vi "stage_control.vi"() -> ()   [LabVIEW 2009]
uses:
  global_stage_initialised.vi
  <vilib>/Utility/inputDevices.llb/joystickAcquire.vi
  <vilib>/Utility/inputDevices.llb/closeJoystick.vi
panel:
  in  "Joystick Index":i32
  in  "SN von Controller 1":string="0135500571"
  in  "Position auslesen":bool
  out "Joystickauslese":T1(ring)
  out "X-Achse pos/neg fahren":i32 min=-3000 max=2000
  out "Y-Achse pos/neg fahren":i32 min=-3000 max=2000
  in  "Schrittweite verringern":bool
  in  "Schrittweite erhoehen":bool
  out "Z-Achse pos fahren":bool
  out "Z-Achse neg fahren":bool
  out "Joystick ID":refnum<k1> caption="Geräte-ID"
  out "z-Achse":i32
  out "y-Achse":i32
  out "x-Achse":i32
  in  "Schrittweite [µm]":u16(ring) items=["500,0", "200,0", "100,0", "50,0", "20,0", "10,0", "5,0", "2,0", "1,0", "0,5", "0,1"]
  out "Aktuelle xyz-Position [mm]":dbl[](array[numeric]) format="%.5g"
  in  "Geschwindigkeit einstellen":bool
  in  "Ziel Geschwindigkeit [mm/s]":dbl=0.3 min=0.01 max=0.6 step=0.001 format="%.3g"
  out "Geschwindigkeit [mm/s]":dbl format="%.3g"
  in  "Negativer Schritt":bool[](array[boolean])
  in  "Positiver Schritt":bool[](array[boolean])
  out "error out":errorcluster
  out "Achse in \nBewegung":bool
  in  "Ziel xyz-Position [mm]":dbl[](array[numeric]) step=1e-05 format="%.5g"
  out "xyz-Bezeichnung":string[](array[string])=["x [mm]", "y [mm]", "z [mm]"]
  in  "Bühnen schließen":bool
  out "Bühnen\ninitialisiert":bool
  # "Steuerung der 3D-Translationsbühne von PI"
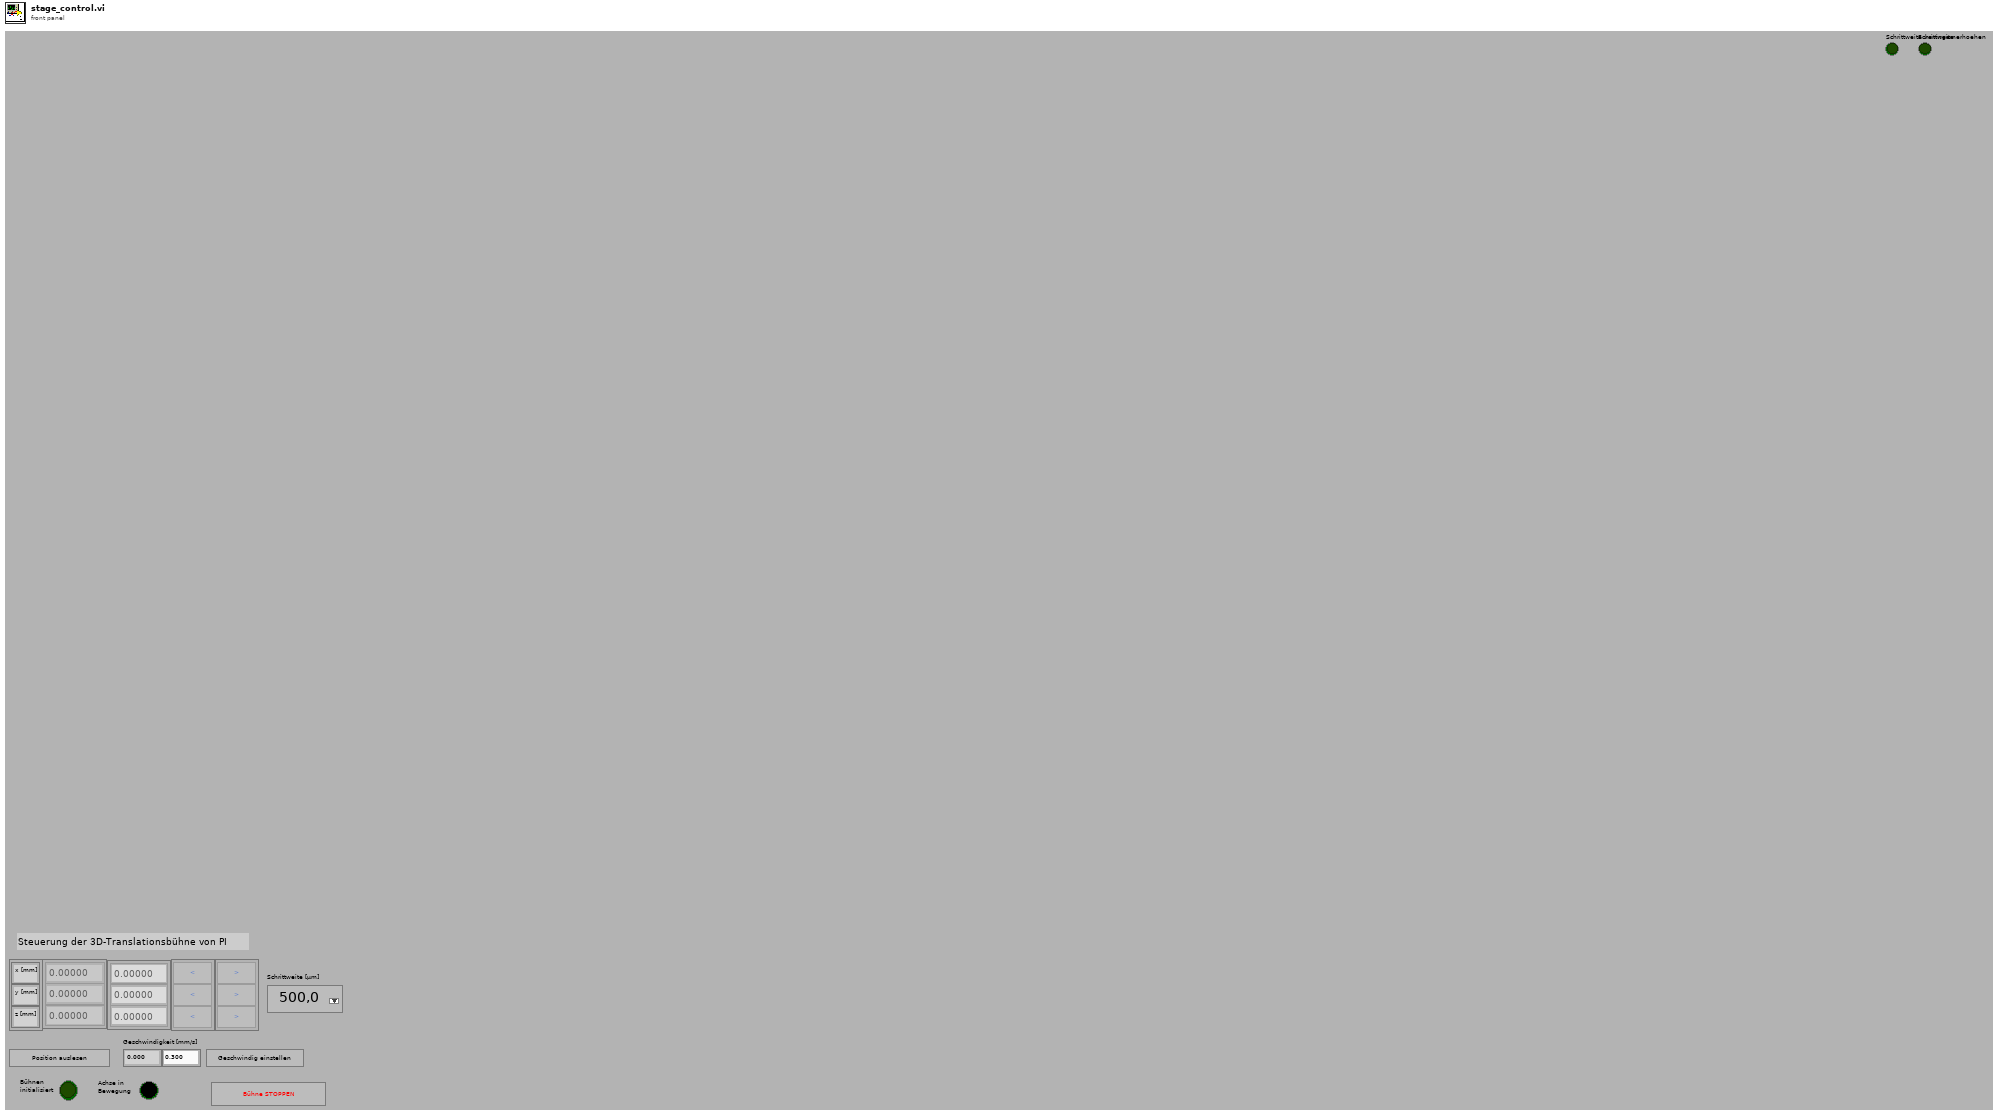
[diagram p1: front panel]
types:
  T1 = enum16{"Nichts tun", "X-Achse", "Y-Achse", "Z-Achse positiv", "Z-Achse negativ", "Schrittweite erhoehen", "Schrittweite verringern"}
  T2 = cluster{"X axis":i32, "Y axis":i32, "Z axis":i32, "X axis rotation":i32, "Y axis rotation":i32, "Z axis rotation":i32, "U axis":i32, "V axis":i32}
  T3 = cluster{"button 1":bool, "button 2":bool, "button 3":bool, "button 4":bool, "button 5":bool, "button 6":bool, "button 7":bool, "button 8":bool, "button 9":bool, "button 10":bool, "button 11":bool, "button 12":bool, "button 13":bool, "button 14":bool, "button 15":bool, "button 16":bool, "button 17":bool, "button 18":bool, "button 19":bool, "button 20":bool, "button 21":bool, "button 22":bool, "button 23":bool, "button 24":bool, "button 25":bool, "button 26":bool, "button 27":bool, "button 28":bool, "button 29":bool, "button 30":bool, "button 31":bool, "button 32":bool}
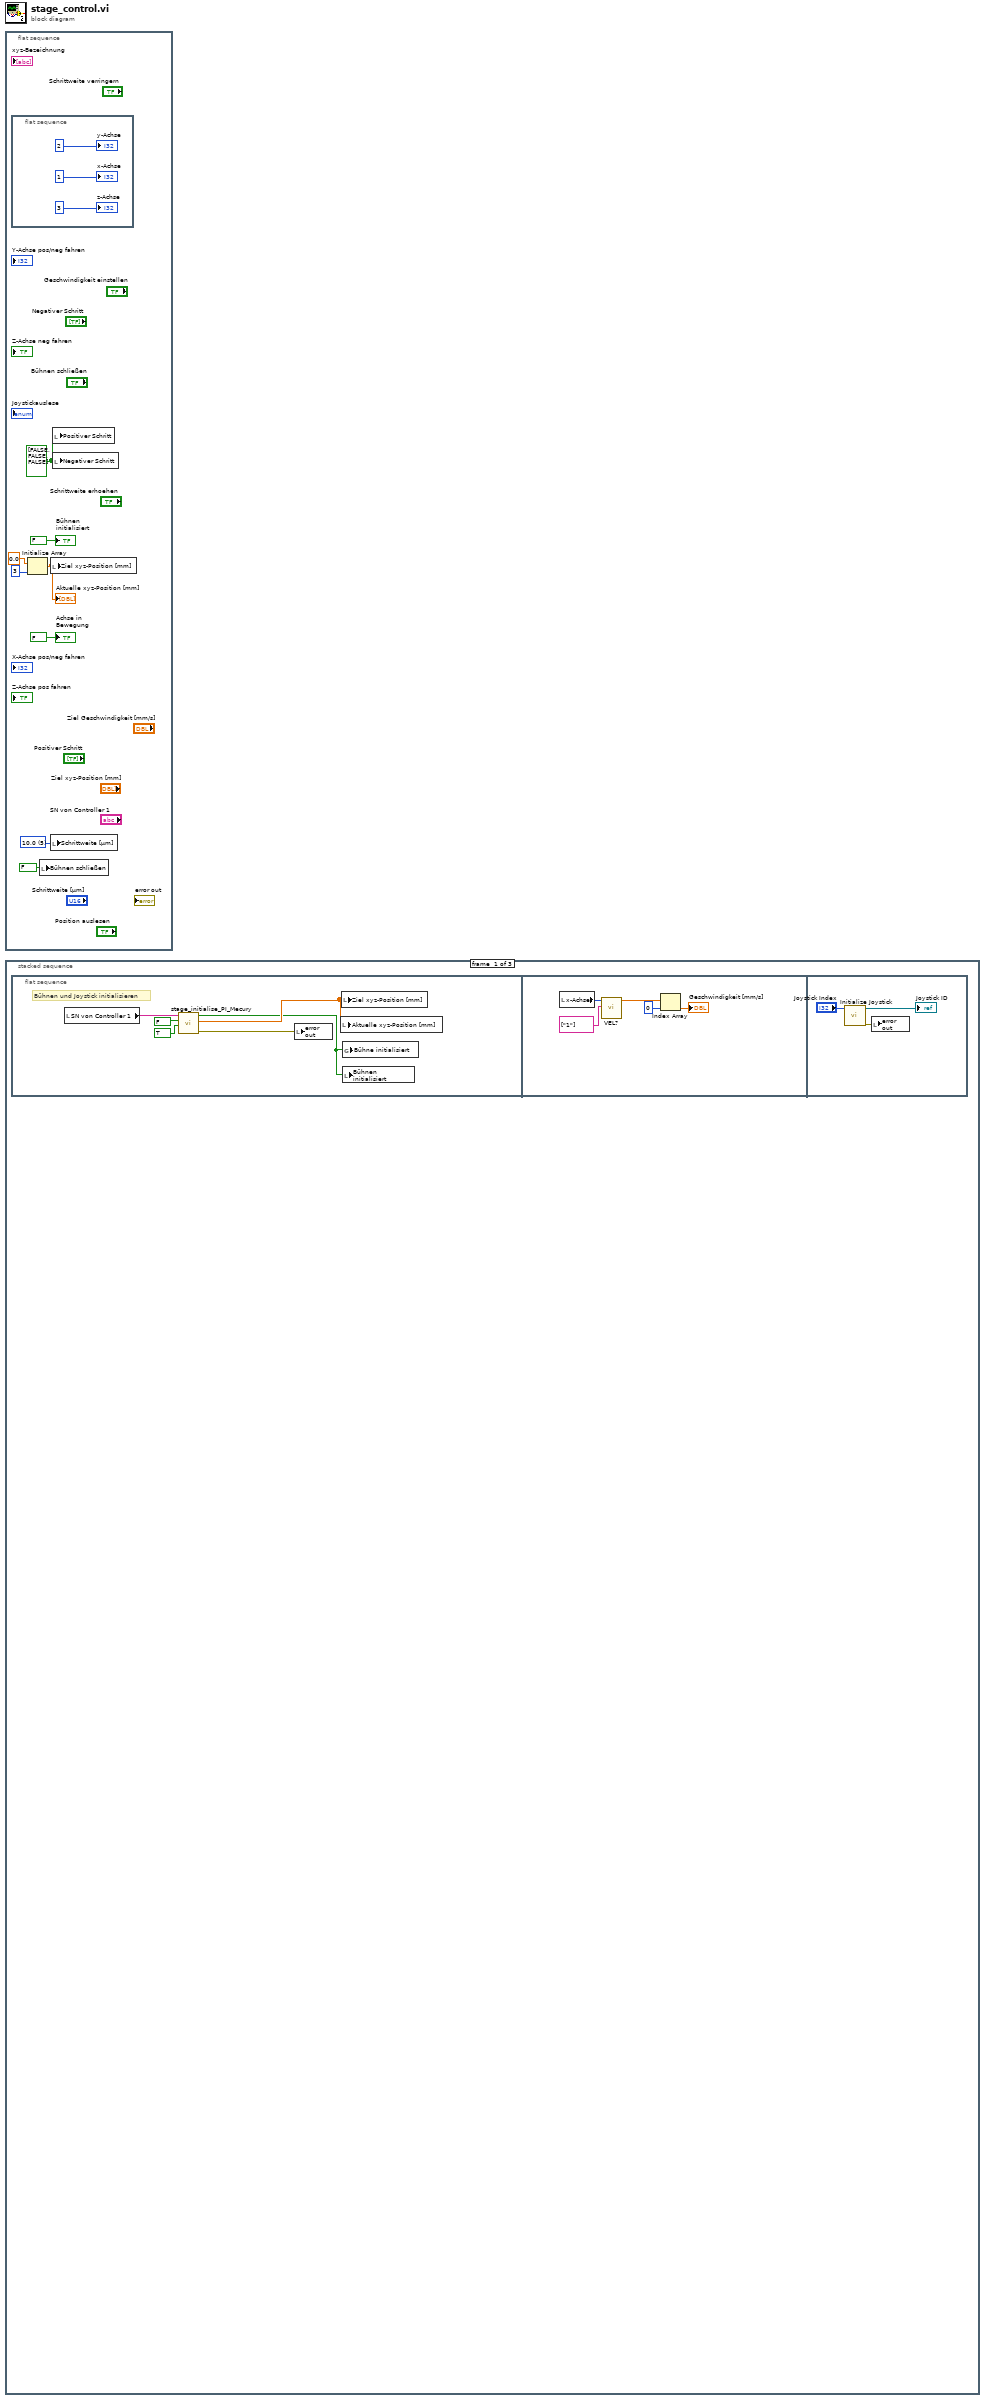
[diagram p0: block diagram]
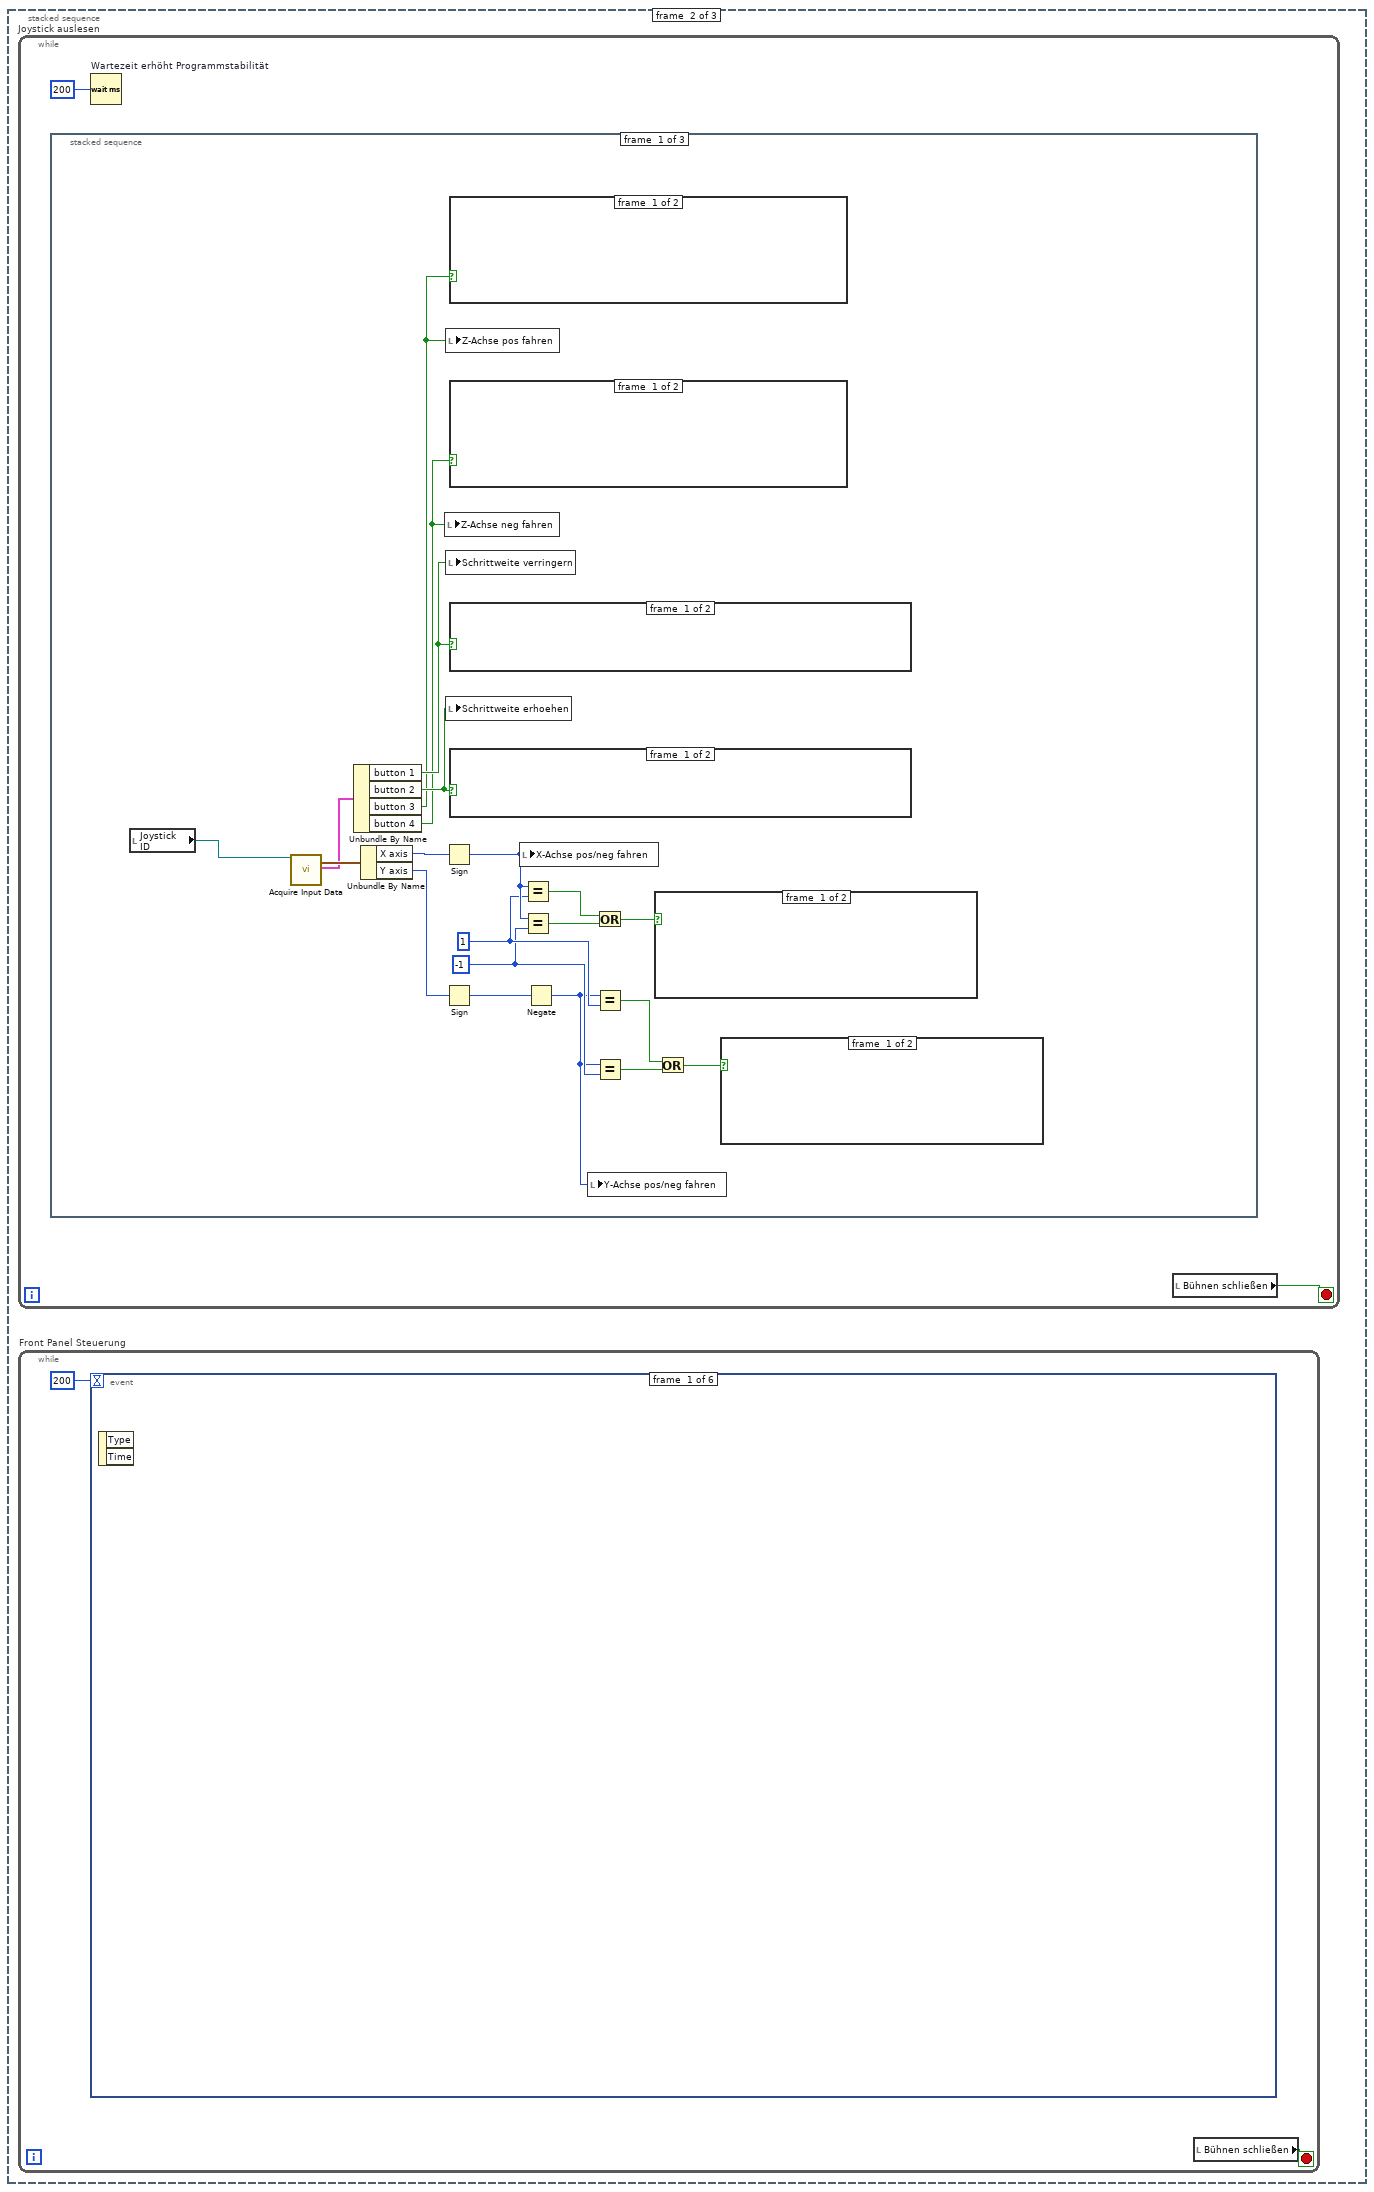
[diagram p2: hidden frame]
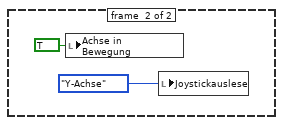
[diagram p3: hidden frame]
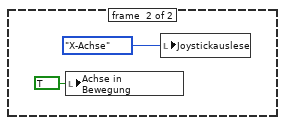
[diagram p4: hidden frame]
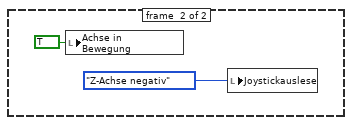
[diagram p5: hidden frame]
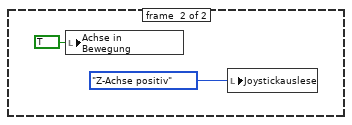
[diagram p6: hidden frame]
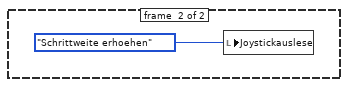
[diagram p7: hidden frame]
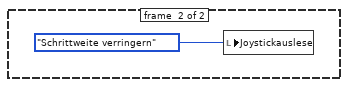
[diagram p8: hidden frame]
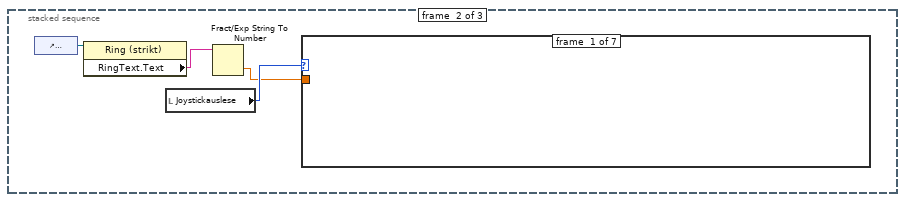
[diagram p9: hidden frame]
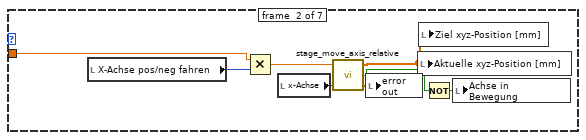
[diagram p10: hidden frame]
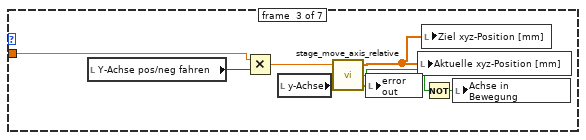
[diagram p11: hidden frame]
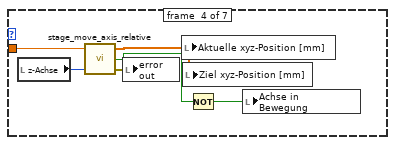
[diagram p12: hidden frame]
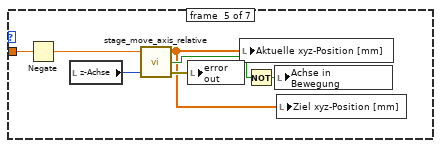
[diagram p13: hidden frame]
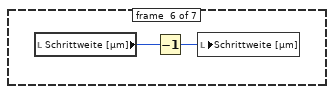
[diagram p14: hidden frame]
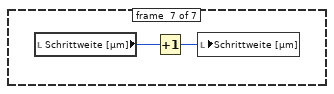
[diagram p15: hidden frame]
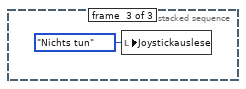
[diagram p16: hidden frame]
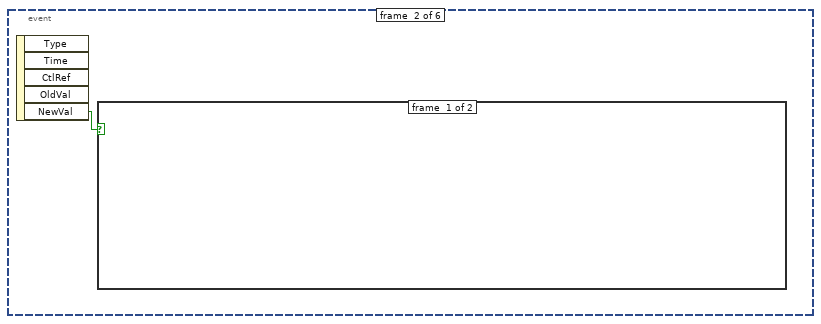
[diagram p17: hidden frame]
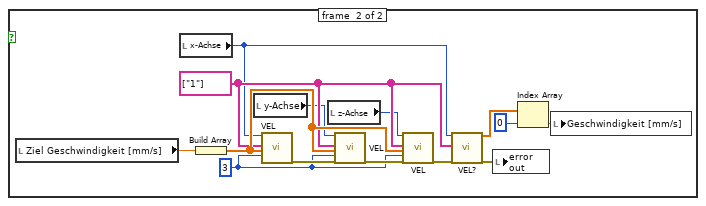
[diagram p18: hidden frame]
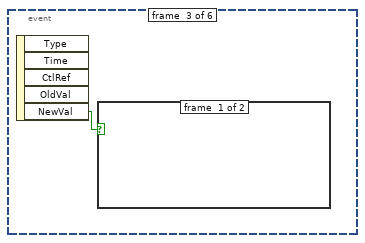
[diagram p19: hidden frame]
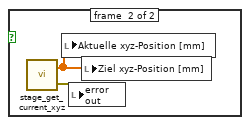
[diagram p20: hidden frame]
diagram:
  n1 = flat-sequence {
    frame #0 {
      w7 = u16 5 items=["500,0", "200,0", "100,0", "50,0", "20,0", "10,0", "5,0", "2,0", "1,0", "0,5"] ("Schrittweite [µm]")
      w3 = bool[] [FALSE, FALSE, FALSE] ("Positiver Schritt")
      n2 = flat-sequence {
        frame #0 {
          "x-Achse" <- 1 ("x-Achse")
          "y-Achse" <- 2 ("y-Achse")
          "z-Achse" <- 3 ("z-Achse")
        }
      }
      n3 = Initialize Array(0.0 ("Element"), 3 ("Dimension")) -> (w6:dbl[])
      "Aktuelle xyz-Position [mm]" <- w6
      n4 = local write "Bühnen schließen"(FALSE ("Bühnen schließen")) -> ()
      n5 = local write "Schrittweite [µm]"(w7) -> ()
      n6 = local write "Ziel xyz-Position [mm]"(w6) -> ()
      n7 = local write "Positiver Schritt"(w3) -> ()
      n8 = local write "Negativer Schritt"(w3) -> ()
      "Bühnen\ninitialisiert" <- FALSE ("Bühnen initialisiert")
      "Achse in \nBewegung" <- FALSE ("x-Achse in Bewegung")
    }
  }
  n9 = stacked-sequence {
    frame #0 {
      n10 = flat-sequence {
        frame #0 {
          # "Bühnen und Joystick initialisieren"
          n11 = local read "SN von Controller 1"() -> (w12:string)
          n12 = call "stage_initialise_PI_Mecury.vi"("Referenz Modus"=TRUE, "Referenzierung erzwingen"=FALSE, "SN von Controller 1"=w12) -> ("error out"=w15:errorcluster, "Aktuelle xyz-Position"=w14:dbl[], "Bühnen initialisiert"=w13:bool)  [unwired: 6 in]
          n13 = local write "error out"(w15) -> ()
          n14 = local write "Aktuelle xyz-Position [mm]"(w14) -> ()
          n15 = local write "Ziel xyz-Position [mm]"(w14) -> ()
          n16 = local write "Bühnen\ninitialisiert"(w13) -> ()
          n17 = global write "global_stage_initialised.vi" "Bühne initialisiert"(w13) -> ()
        }
        frame #1 {
          n18 = local read "x-Achse"() -> (w18:i32)
          n19 = call "VEL?.vi"("System no."=w18, "Axes to query"=string[] ["1"]) -> ("Velocity"=w19:dbl[])  [unwired: 16 in, 1 out]
          n20 = Index Array(array=w19, index=0 ("Index")) -> (element=→"Geschwindigkeit [mm/s]":dbl)
        }
        frame #2 {
          n21 = call <vilib>:"Initialize Joystick.vi"("device index"="Joystick Index") -> ("error out"=w24:errorcluster, "device ID"=→"Joystick ID":refnum<k1>)  [unwired: 9 in]
          n22 = local write "error out"(w24) -> ()
        }
      }
    }
    frame #1 {
      n23 = while "Joystick auslesen" {
        stop <- w27 stop-if-true
        n24 = stacked-sequence {
          frame #0 {
            w32 = -1
            w33 = 1
            n25 = local read "Joystick ID"() -> (w47:refnum<k1>)
            n26 = call-poly <vilib>:"Acquire Input Data.vi"("device ID"=w47) -> ("axis info"=w46:T2, "button info"=w45:T3)  [unwired: 14 in, 3 out]
            n27 = Unbundle By Name(w45) -> ("button 1"=w41:bool, "button 2"=w40:bool, "button 3"=w39:bool, "button 4"=w38:bool)
            n28 = Unbundle By Name(w46) -> ("X axis"=w44:i32, "Y axis"=w42:i32)
            n29 = Sign(1:w44) -> (0:w34:i32)
            n30 = Sign(1:w42) -> (0:w43:i32)
            n31 = local write "Z-Achse neg fahren"(w38) -> ()
            n32 = local write "Z-Achse pos fahren"(w39) -> ()
            n33 = local write "Schrittweite verringern"(w41) -> ()
            n34 = local write "Schrittweite erhoehen"(w40) -> ()
            n35 = case shown="True" w39 {
              frame #0 {
              }
              frame #1 {
                n36 = local write "Achse in \nBewegung"(TRUE ("Achse in Bewegung")) -> ()
                n37 = local write "Joystickauslese"(T1."Z-Achse positiv" ("Joystickauslese")) -> ()
              }
            }
            n38 = case shown="True" w38 {
              frame #0 {
              }
              frame #1 {
                n39 = local write "Achse in \nBewegung"(TRUE ("Achse in Bewegung")) -> ()
                n40 = local write "Joystickauslese"(T1."Z-Achse negativ" ("Joystickauslese")) -> ()
              }
            }
            n41 = case shown="True" w41 {
              frame #0 {
              }
              frame #1 {
                n42 = local write "Joystickauslese"(T1."Schrittweite verringern" ("Joystickauslese")) -> ()
              }
            }
            n43 = case shown="True" w40 {
              frame #0 {
              }
              frame #1 {
                n44 = local write "Joystickauslese"(T1."Schrittweite erhoehen" ("Joystickauslese")) -> ()
              }
            }
            n45 = local write "X-Achse pos/neg fahren"(w34) -> ()
            n46 = Equal?(x=w34, y=w33) -> (x = y?=w37:bool)
            n47 = Equal?(x=w34, y=w32) -> (x = y?=w36:bool)
            n48 = Negate(x=w43) -> (-x=w29:i32)
            n49 = local write "Y-Achse pos/neg fahren"(w29) -> ()
            n50 = Or(x=w37, y=w36) -> (x .or. y?=w35:bool)
            n51 = Equal?(x=w29, y=w33) -> (x = y?=w30:bool)
            n52 = Equal?(x=w29, y=w32) -> (x = y?=w31:bool)
            n53 = case shown="True" w35 {
              frame #0 {
              }
              frame #1 {
                n54 = local write "Achse in \nBewegung"(TRUE ("Achse in Bewegung")) -> ()
                n55 = local write "Joystickauslese"(T1."X-Achse" ("Joystickauslese")) -> ()
              }
            }
            n56 = Or(x=w30, y=w31) -> (x .or. y?=w28:bool)
            n57 = case shown="True" w28 {
              frame #0 {
              }
              frame #1 {
                n58 = local write "Achse in \nBewegung"(TRUE ("Achse in Bewegung")) -> ()
                n59 = local write "Joystickauslese"(T1."Y-Achse" ("Joystickauslese")) -> ()
              }
            }
          }
          frame #1 {
            n60 = control-ref of="Schrittweite [µm]"() -> (w59:refnum<vi>)
            n61 = property class="Ring (strikt)"(reference=w59) -> ("RingText.Text"=w60:string)  [unwired: 1 in, 2 out]
            n62 = local read "Joystickauslese"() -> (w61:T1)
            n63 = Fract/Exp String To Number(string=w60) -> (number=w58:dbl)  [unwired: 3 in, 1 out]
            n64 = case shown="\"X-Achse\"" w61 {
              tunnel: w58 -> [_ w64 w75 w80 w87 _ _]
              frame #0 {
              }
              frame #1 {
                n65 = local read "X-Achse pos/neg fahren"() -> (w67:i32)
                n66 = Multiply(x=w64, y=w67) -> (x*y=w66:dbl)
                n67 = local read "x-Achse"() -> (w65:i32)
                n68 = call "stage_move_axis_relative.vi"("Achse"=w65, "Schrittweite [µm]"=w66) -> ("error out"=w69:errorcluster, "Fertig?"=w68:bool, "xyz-Position OUT [mm]"=w62:dbl[])  [unwired: 1 in]
                n69 = local write "error out"(w69) -> ()
                n70 = local write "Aktuelle xyz-Position [mm]"(w62) -> ()
                n71 = local write "Ziel xyz-Position [mm]"(w62) -> ()
                n72 = Not(x=w68) -> (.not. x?=w63:bool)
                n73 = local write "Achse in \nBewegung"(w63) -> ()
              }
              frame #2 {
                n74 = local read "Y-Achse pos/neg fahren"() -> (w74:i32)
                n75 = Multiply(x=w75, y=w74) -> (x*y=w73:dbl)
                n76 = local read "y-Achse"() -> (w72:i32)
                n77 = call "stage_move_axis_relative.vi"("Achse"=w72, "Schrittweite [µm]"=w73) -> ("error out"=w77:errorcluster, "Fertig?"=w76:bool, "xyz-Position OUT [mm]"=w70:dbl[])  [unwired: 1 in]
                n78 = local write "error out"(w77) -> ()
                n79 = local write "Aktuelle xyz-Position [mm]"(w70) -> ()
                n80 = local write "Ziel xyz-Position [mm]"(w70) -> ()
                n81 = Not(x=w76) -> (.not. x?=w71:bool)
                n82 = local write "Achse in \nBewegung"(w71) -> ()
              }
              frame #3 {
                n83 = local read "z-Achse"() -> (w81:i32)
                n84 = call "stage_move_axis_relative.vi"("Achse"=w81, "Schrittweite [µm]"=w80) -> ("error out"=w83:errorcluster, "Fertig?"=w82:bool, "xyz-Position OUT [mm]"=w78:dbl[])  [unwired: 1 in]
                n85 = local write "error out"(w83) -> ()
                n86 = local write "Aktuelle xyz-Position [mm]"(w78) -> ()
                n87 = local write "Ziel xyz-Position [mm]"(w78) -> ()
                n88 = Not(x=w82) -> (.not. x?=w79:bool)
                n89 = local write "Achse in \nBewegung"(w79) -> ()
              }
              frame #4 {
                n90 = Negate(x=w87) -> (-x=w86:dbl)
                n91 = local read "z-Achse"() -> (w88:i32)
                n92 = call "stage_move_axis_relative.vi"("Achse"=w88, "Schrittweite [µm]"=w86) -> ("error out"=w90:errorcluster, "Fertig?"=w89:bool, "xyz-Position OUT [mm]"=w84:dbl[])  [unwired: 1 in]
                n93 = local write "error out"(w90) -> ()
                n94 = local write "Aktuelle xyz-Position [mm]"(w84) -> ()
                n95 = Not(x=w89) -> (.not. x?=w85:bool)
                n96 = local write "Achse in \nBewegung"(w85) -> ()
                n97 = local write "Ziel xyz-Position [mm]"(w84) -> ()
              }
              frame #5 {
                n98 = local read "Schrittweite [µm]"() -> (w91:u16)
                n99 = Decrement(x=w91) -> (x-1=w92:u16)
                n100 = local write "Schrittweite [µm]"(w92) -> ()
              }
              frame #6 {
                n101 = local read "Schrittweite [µm]"() -> (w94:u16)
                n102 = Increment(x=w94) -> (x+1=w93:u16)
                n103 = local write "Schrittweite [µm]"(w93) -> ()
              }
            }
          }
          frame #2 {
            n104 = local write "Joystickauslese"(T1."Nichts tun" ("Joystickauslese")) -> ()
          }
        }
        n105 = Wait (ms) "Wartezeit erhöht Programmstabilität"(milliseconds to wait=u32 200 ("Zu wartende ms")) -> ()  [unwired: 1 out]
        n106 = local read "Bühnen schließen"() -> (w27:bool)
      }
      n107 = while "Front Panel Steuerung" {
        stop <- w96 stop-if-true
        n108 = event shown="[3] \"Ziel xyz-Position [mm]\": Wertänderung" {
          selector: _ -> [_ _ _ _ _ _]
          dyn-events: _ -> [_ _ _ _ _ _]
          timeout: 200 -> [_ _ _ _ _ _]
          event #0 {
            n109 = event-data() -> ()  [unwired: 1 in, 2 out]
          }
          event #1 {
            n110 = event-data() -> ("NewVal"=w98:bool)  [unwired: 1 in, 4 out]
            n111 = case shown="True" w98 {
              frame #0 {
              }
              frame #1 {
                w109 = i16 3 ("No.of digits")
                w105 = string[] ["1"] ("Axes to set")
                n112 = local read "Ziel Geschwindigkeit [mm/s]"() -> (w110:dbl)
                n113 = local read "x-Achse"() -> (w101:i32)
                n114 = Build Array(w110) -> (w108:dbl[])
                n115 = local read "y-Achse"() -> (w100:i32)
                n116 = call "VEL.vi"("System no."=w101, "Axes to set"=w105, "Velocity values"=w108, "No.of digits"=w109) -> ("error out"=w112:errorcluster)  [unwired: 14 in, 1 out]
                n117 = local read "z-Achse"() -> (w99:i32)
                n118 = call "VEL.vi"("System no."=w100, "Axes to set"=w105, "Velocity values"=w108, "No.of digits"=w109, "error in"=w112) -> ("error out"=w111:errorcluster)  [unwired: 13 in, 1 out]
                n119 = call "VEL.vi"("System no."=w99, "Axes to set"=w105, "Velocity values"=w108, "No.of digits"=w109, "error in"=w111) -> ("error out"=w106:errorcluster)  [unwired: 13 in, 1 out]
                n120 = call "VEL?.vi"("System no."=w101, "Axes to query"=w105, "error in"=w106) -> ("Velocity"=w103:dbl[], "error out"=w107:errorcluster)  [unwired: 15 in]
                n121 = local write "error out"(w107) -> ()
                n122 = Index Array(array=w103, index=0 ("Index")) -> (element=w104:dbl)
                n123 = local write "Geschwindigkeit [mm/s]"(w104) -> ()
              }
            }
          }
          event #2 {
            n124 = event-data() -> ("NewVal"=w113:bool)  [unwired: 1 in, 4 out]
            n125 = case shown="True" w113 {
              frame #0 {
              }
              frame #1 {
                n126 = call "stage_get_current_xyz.vi"() -> ("error out"=w115:errorcluster, "Aktuelle xyz-Position OUT [mm]"=w114:dbl[])  [unwired: 3 in]
                n127 = local write "Aktuelle xyz-Position [mm]"(w114) -> ()
                n128 = local write "error out"(w115) -> ()
                n129 = local write "Ziel xyz-Position [mm]"(w114) -> ()
              }
            }
          }
          event #3 {
            n130 = event-data() -> ("OldVal"=w117:dbl[], "NewVal"=w116:dbl[])  [unwired: 1 in, 3 out]
            n131 = flat-sequence {
              tunnel: [w123] -> w120
              tunnel: [w122] -> w119
              tunnel: [w121] -> w118
              tunnel: w117 -> [w125]
              tunnel: w116 -> [w124]
              tunnel: w120 -> [w139]
              tunnel: w119 -> [w138]
              tunnel: w118 -> [w137]
              frame #0 {
                w128 = 2 ("Index")
                w127 = 1 ("Index")
                w126 = 0 ("Index")
                # "Änderung des Ziels: Entscheide welche Achse gefahren werden soll"
                n132 = local write "Achse in \nBewegung"(TRUE ("x-Achse in Bewegung")) -> ()
                n133 = Index Array(array=w125, index #1=w126, index #2=w127, index #3=w128) -> (element #1=w129:dbl, element #2=w130:dbl, element #3=w133:dbl)
                n134 = Index Array(array=w124, index #1=w126, index #2=w127, index #3=w128) -> (element #1=w134:dbl, element #2=w131:dbl, element #3=w132:dbl)
                n135 = Not Equal?(x=w129, y=w134) -> (x != y?=w123:bool)
                n136 = Not Equal?(x=w130, y=w131) -> (x != y?=w122:bool)
                n137 = Not Equal?(x=w133, y=w132) -> (x != y?=w121:bool)
              }
              frame #1 {
                n138 = local read "Ziel xyz-Position [mm]"() -> (w136:dbl[])
                n139 = case shown="True" w139 {
                  tunnel: w136 -> [_ w156]
                  frame #0 {
                  }
                  frame #1 {
                    n140 = local read "x-Achse"() -> (w154:i32)
                    n141 = call "stage_move_axis_absolute.vi"("Ziel xyz IN [mm]"=w156, "Achse"=w154) -> ("error out"=w157:errorcluster, "Fertig?"=w155:bool, "Ziel xyz OUT [mm]"=w152:dbl[])  [unwired: 1 in]
                    n142 = local write "Aktuelle xyz-Position [mm]"(w152) -> ()
                    n143 = local write "Ziel xyz-Position [mm]"(w152) -> ()
                    n144 = local write "error out"(w157) -> ()
                    n145 = Not(x=w155) -> (.not. x?=w153:bool)
                    n146 = local write "Achse in \nBewegung"(w153) -> ()
                  }
                }
                n147 = case shown="True" w138 {
                  tunnel: w136 -> [_ w150]
                  frame #0 {
                  }
                  frame #1 {
                    n148 = local read "y-Achse"() -> (w148:i32)
                    n149 = call "stage_move_axis_absolute.vi"("Ziel xyz IN [mm]"=w150, "Achse"=w148) -> ("error out"=w151:errorcluster, "Fertig?"=w149:bool, "Ziel xyz OUT [mm]"=w146:dbl[])  [unwired: 1 in]
                    n150 = local write "Aktuelle xyz-Position [mm]"(w146) -> ()
                    n151 = local write "Ziel xyz-Position [mm]"(w146) -> ()
                    n152 = local write "error out"(w151) -> ()
                    n153 = Not(x=w149) -> (.not. x?=w147:bool)
                    n154 = local write "Achse in \nBewegung"(w147) -> ()
                  }
                }
                n155 = case shown="True" w137 {
                  tunnel: w136 -> [_ w143]
                  frame #0 {
                  }
                  frame #1 {
                    n156 = local read "z-Achse"() -> (w142:i32)
                    n157 = call "stage_move_axis_absolute.vi"("Ziel xyz IN [mm]"=w143, "Achse"=w142) -> ("error out"=w145:errorcluster, "Fertig?"=w144:bool, "Ziel xyz OUT [mm]"=w140:dbl[])  [unwired: 1 in]
                    n158 = local write "Aktuelle xyz-Position [mm]"(w140) -> ()
                    n159 = local write "Ziel xyz-Position [mm]"(w140) -> ()
                    n160 = local write "error out"(w145) -> ()
                    n161 = Not(x=w144) -> (.not. x?=w141:bool)
                    n162 = local write "Achse in \nBewegung"(w141) -> ()
                  }
                }
              }
            }
          }
          event #4 {
            n163 = event-data() -> ("NewVal"=w162:bool[])  [unwired: 1 in, 4 out]
            n164 = Index Array(array=w162, index #1=0 ("Index"), index #2=1 ("Index"), index #3=2 ("Index")) -> (element #1=w160:bool, element #2=w159:bool, element #3=w158:bool)
            n165 = Compound Arithmetic op=OR(w160, w159, w158) -> (w161:bool)
            n166 = case shown="True" w161 {
              tunnel: w160 -> [_ w168]
              tunnel: w159 -> [_ w167]
              tunnel: w158 -> [_ w166]
              frame #0 {
              }
              frame #1 {
                n167 = flat-sequence {
                  tunnel: [w171] -> w169
                  tunnel: w169 -> [w177]
                  tunnel: w168 -> [w176]
                  tunnel: w167 -> [w175]
                  tunnel: w166 -> [w174]
                  frame #0 {
                    n168 = local write "Achse in \nBewegung"(TRUE ("Achse in Bewegung")) -> ()
                    n169 = control-ref of="Schrittweite [µm]"() -> (w173:refnum<vi>)
                    n170 = property class="Ring (strikt)"(reference=w173) -> ("RingText.Text"=w172:string)  [unwired: 1 in, 2 out]
                    n171 = Fract/Exp String To Number(string=w172) -> (number=w171:dbl)  [unwired: 3 in, 1 out]
                  }
                  frame #1 {
                    n172 = local read "x-Achse"() -> (w180:i32)
                    n173 = local read "y-Achse"() -> (w178:i32)
                    n174 = local read "z-Achse"() -> (w179:i32)
                    n175 = case shown="True" w174 {
                      tunnel: w179 -> [_ w186]
                      tunnel: w177 -> [_ w182]
                      frame #0 {
                      }
                      frame #1 {
                        n176 = call "stage_move_axis_relative.vi"("Achse"=w186, "Schrittweite [µm]"=w182) -> ("error out"=w185:errorcluster, "Fertig?"=w184:bool, "xyz-Position OUT [mm]"=w181:dbl[])  [unwired: 1 in]
                        n177 = local write "Aktuelle xyz-Position [mm]"(w181) -> ()
                        n178 = local write "Ziel xyz-Position [mm]"(w181) -> ()
                        n179 = local write "error out"(w185) -> ()
                        n180 = Not(x=w184) -> (.not. x?=w183:bool)
                        n181 = local write "Achse in \nBewegung"(w183) -> ()
                      }
                    }
                    n182 = case shown="True" w175 {
                      tunnel: w178 -> [_ w191]
                      tunnel: w177 -> [_ w188]
                      frame #0 {
                      }
                      frame #1 {
                        n183 = call "stage_move_axis_relative.vi"("Achse"=w191, "Schrittweite [µm]"=w188) -> ("error out"=w192:errorcluster, "Fertig?"=w190:bool, "xyz-Position OUT [mm]"=w187:dbl[])  [unwired: 1 in]
                        n184 = local write "Aktuelle xyz-Position [mm]"(w187) -> ()
                        n185 = local write "Ziel xyz-Position [mm]"(w187) -> ()
                        n186 = local write "error out"(w192) -> ()
                        n187 = Not(x=w190) -> (.not. x?=w189:bool)
                        n188 = local write "Achse in \nBewegung"(w189) -> ()
                      }
                    }
                    n189 = case shown="True" w176 {
                      tunnel: w180 -> [_ w197]
                      tunnel: w177 -> [_ w194]
                      frame #0 {
                      }
                      frame #1 {
                        n190 = call "stage_move_axis_relative.vi"("Achse"=w197, "Schrittweite [µm]"=w194) -> ("error out"=w198:errorcluster, "Fertig?"=w196:bool, "xyz-Position OUT [mm]"=w193:dbl[])  [unwired: 1 in]
                        n191 = local write "Aktuelle xyz-Position [mm]"(w193) -> ()
                        n192 = local write "Ziel xyz-Position [mm]"(w193) -> ()
                        n193 = local write "error out"(w198) -> ()
                        n194 = Not(x=w196) -> (.not. x?=w195:bool)
                        n195 = local write "Achse in \nBewegung"(w195) -> ()
                      }
                    }
                  }
                }
              }
            }
          }
          event #5 {
            n196 = event-data() -> ("NewVal"=w203:bool[])  [unwired: 1 in, 4 out]
            n197 = Index Array(array=w203, index #1=0 ("Index"), index #2=1 ("Index"), index #3=2 ("Index")) -> (element #1=w201:bool, element #2=w200:bool, element #3=w199:bool)
            n198 = Compound Arithmetic op=OR(w201, w200, w199) -> (w202:bool)
            n199 = case shown="True" w202 {
              tunnel: w201 -> [_ w209]
              tunnel: w200 -> [_ w208]
              tunnel: w199 -> [_ w207]
              frame #0 {
              }
              frame #1 {
                n200 = flat-sequence {
                  tunnel: [w213] -> w210
                  tunnel: w210 -> [w219]
                  tunnel: w209 -> [w218]
                  tunnel: w208 -> [w217]
                  tunnel: w207 -> [w216]
                  frame #0 {
                    n201 = local write "Achse in \nBewegung"(TRUE ("Achse in Bewegung")) -> ()
                    n202 = control-ref of="Schrittweite [µm]"() -> (w215:refnum<vi>)
                    n203 = property class="Ring (strikt)"(reference=w215) -> ("RingText.Text"=w214:string)  [unwired: 1 in, 2 out]
                    n204 = Fract/Exp String To Number(string=w214) -> (number=w212:dbl)  [unwired: 3 in, 1 out]
                    n205 = Negate(x=w212) -> (-x=w213:dbl)
                  }
                  frame #1 {
                    n206 = local read "x-Achse"() -> (w220:i32)
                    n207 = local read "y-Achse"() -> (w221:i32)
                    n208 = local read "z-Achse"() -> (w222:i32)
                    n209 = case shown="True" w216 {
                      tunnel: w222 -> [_ w228]
                      tunnel: w219 -> [_ w224]
                      frame #0 {
                      }
                      frame #1 {
                        n210 = call "stage_move_axis_relative.vi"("Achse"=w228, "Schrittweite [µm]"=w224) -> ("error out"=w227:errorcluster, "Fertig?"=w226:bool, "xyz-Position OUT [mm]"=w223:dbl[])  [unwired: 1 in]
                        n211 = local write "Aktuelle xyz-Position [mm]"(w223) -> ()
                        n212 = local write "Ziel xyz-Position [mm]"(w223) -> ()
                        n213 = local write "error out"(w227) -> ()
                        n214 = Not(x=w226) -> (.not. x?=w225:bool)
                        n215 = local write "Achse in \nBewegung"(w225) -> ()
                      }
                    }
                    n216 = case shown="True" w217 {
                      tunnel: w221 -> [_ w233]
                      tunnel: w219 -> [_ w230]
                      frame #0 {
                      }
                      frame #1 {
                        n217 = call "stage_move_axis_relative.vi"("Achse"=w233, "Schrittweite [µm]"=w230) -> ("error out"=w234:errorcluster, "Fertig?"=w232:bool, "xyz-Position OUT [mm]"=w229:dbl[])  [unwired: 1 in]
                        n218 = local write "Aktuelle xyz-Position [mm]"(w229) -> ()
                        n219 = local write "Ziel xyz-Position [mm]"(w229) -> ()
                        n220 = local write "error out"(w234) -> ()
                        n221 = Not(x=w232) -> (.not. x?=w231:bool)
                        n222 = local write "Achse in \nBewegung"(w231) -> ()
                      }
                    }
                    n223 = case shown="True" w218 {
                      tunnel: w220 -> [_ w239]
                      tunnel: w219 -> [_ w236]
                      frame #0 {
                      }
                      frame #1 {
                        n224 = call "stage_move_axis_relative.vi"("Achse"=w239, "Schrittweite [µm]"=w236) -> ("error out"=w240:errorcluster, "Fertig?"=w238:bool, "xyz-Position OUT [mm]"=w235:dbl[])  [unwired: 1 in]
                        n225 = local write "Aktuelle xyz-Position [mm]"(w235) -> ()
                        n226 = local write "Ziel xyz-Position [mm]"(w235) -> ()
                        n227 = local write "error out"(w240) -> ()
                        n228 = Not(x=w238) -> (.not. x?=w237:bool)
                        n229 = local write "Achse in \nBewegung"(w237) -> ()
                      }
                    }
                  }
                }
              }
            }
          }
        }
        n230 = local read "Bühnen schließen"() -> (w96:bool)
      }
    }
    frame #2 {
      n231 = flat-sequence {
        frame #0 {
          n232 = local read "Joystick ID"() -> (w241:refnum<k1>)
          n233 = call-poly <vilib>:"Close Input Device.vi"("device ID"=w241) -> ("error out"=w242:errorcluster)  [unwired: 9 in]
          n234 = local write "error out"(w242) -> ()
        }
        frame #1 {
          # "Verbindung zu Bühnen schließen"
          n235 = local read "x-Achse"() -> (w245:i32)
          n236 = call "Close connection if open.vi"("System no."=w245, "Close DaisyChain"=TRUE) -> ("error out"=w249:errorcluster)  [unwired: 16 in, 1 out]
          n237 = local read "y-Achse"() -> (w244:i32)
          n238 = call "Close connection if open.vi"("System no."=w244, "Close DaisyChain"=TRUE, "error in"=w249) -> ("error out"=w250:errorcluster)  [unwired: 15 in, 1 out]
          n239 = local read "z-Achse"() -> (w243:i32)
          n240 = call "Close connection if open.vi"("System no."=w243, "Close DaisyChain"=TRUE, "error in"=w250) -> ("error out"=w247:errorcluster)  [unwired: 15 in, 1 out]
          n241 = local write "error out"(w247) -> ()
          n242 = Unbundle By Name(w247) -> ("status"=w246:bool)
          n243 = local write "Bühnen\ninitialisiert"(w246) -> ()
          n244 = global write "global_stage_initialised.vi" "Bühne initialisiert"(w246) -> ()
        }
      }
    }
  }
